vi "DVR Performance Test v3.vi"() -> ()   [LabVIEW 2021]
uses:
  Source/Support/Nodes/abs_Node/Status.ctl
  Source/Support/Nodes/abs_Node/bt_Node.lvclass
panel:
  out "x-y":dbl format="%#_6p"
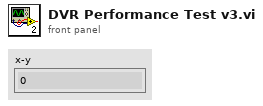
[diagram p1: front panel]
types:
  T1 = typedef "BT.lvlib/bt_Node.lvclass/Status.ctl" = enum16{"Success", "Failure", "Running"}
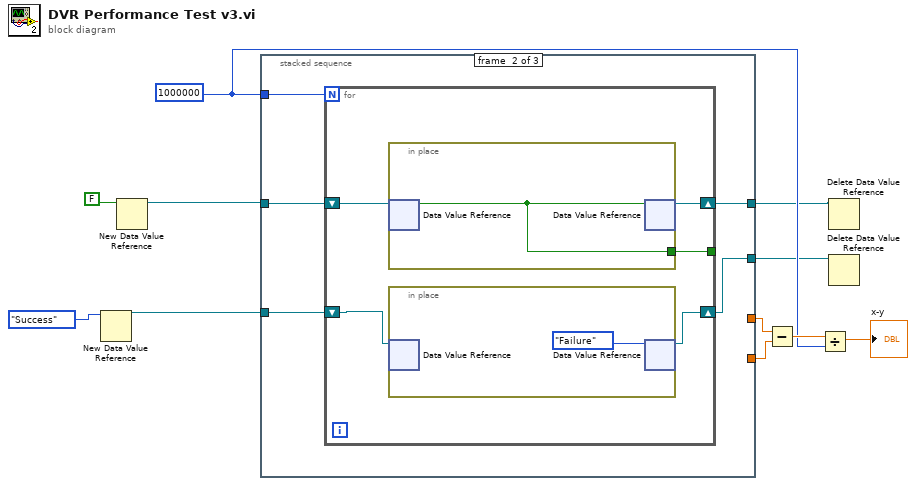
[diagram p0: block diagram]
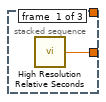
[diagram p2: hidden frame]
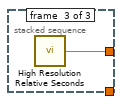
[diagram p3: hidden frame]
diagram:
  w7 = 1000000
  n1 = New Data Value Reference(data value=Status."Success" ("Status")) -> (data value reference=w3:refnum<data-value>)  [unwired: 1 in, 1 out]
  n2 = New Data Value Reference(data value=FALSE) -> (data value reference=w6:refnum<data-value>)  [unwired: 1 in, 1 out]
  n3 = stacked-sequence {
    tunnel: w6 -> [_ w17 _]
    tunnel: [_ w16 _] -> w4
    tunnel: [w12 _ _] -> w11
    tunnel: [_ _ w25] -> w10
    tunnel: w7 -> [_ w15 _]
    tunnel: w3 -> [_ w14 _]
    tunnel: [_ w13 _] -> w2
    frame #0 {
      n4 = call <vilib>:"High Resolution Relative Seconds.vi"() -> ("relative seconds"=w12:dbl)
    }
    frame #1 {
      n5 = for {
        N: w15 -> [_]
        shift-right: [w21] -> w16
        shift-left: w17 -> [w22]
        tunnel: [w20] -> _
        shift-right: [w18] -> w13
        shift-left: w14 -> [w19]
        n6 = in-place {
          in-place-border: [w24] -> w20
          n7 = in-place-dvr #1(w22) -> (w24:bool)  [unwired: 1 out]
          n8 = in-place-dvr #1(w24) -> (w21:refnum<data-value>)  [unwired: 1 out]
        }
        n9 = in-place {
          n10 = in-place-dvr #2(w19) -> ()  [unwired: 2 out]
          n11 = in-place-dvr #2(Status."Failure" ("Status")) -> (w18:refnum<data-value>)  [unwired: 1 out]
        }
      }
    }
    frame #2 {
      n12 = call <vilib>:"High Resolution Relative Seconds.vi"() -> ("relative seconds"=w25:dbl)
    }
  }
  n13 = Subtract(x=w10, y=w11) -> (x-y=w9:dbl)
  n14 = Divide(x=w9, y=w7) -> (x/y=→"x-y":dbl)
  n15 = Delete Data Value Reference(data value reference=w4) -> ()  [unwired: 1 in, 2 out]
  n16 = Delete Data Value Reference(data value reference=w2) -> ()  [unwired: 1 in, 2 out]
